vi "Shutdown.vi"(8 "error in (no error)":errorcluster, 11 "Stage_MadCityLabMicro in":refnum<class "Stage_MadCityLabMicro.lvclass">) -> (0 "error out":errorcluster, 3 "Stage_MadCityLabMicro out":refnum<class "Stage_MadCityLabMicro.lvclass">)   [LabVIEW 2020, in "Stage_MadCityLabMicro.lvlib" / "Stage_MadCityLabMicro.lvclass"]
uses:
  Stage_MadCityLabMicro.lvclass
  Stage_MadCityLabMicro.lvclass/Stage_MadCityLabMicro.ctl
  Hardware Abstraction Layer/Component/Stage/Stage/Stage.lvclass
  Dependency/MicroDrive.dll
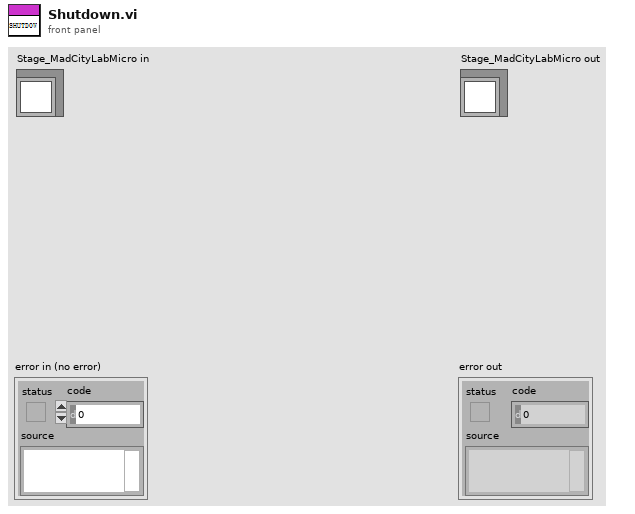
[diagram p1: front panel]
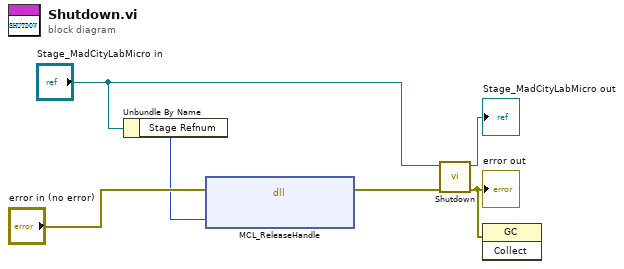
[diagram p0: block diagram]
diagram:
  n1 = Unbundle By Name("Stage_MadCityLabMicro in") -> ("Stage Refnum"=w1:i32)
  n2 = dll-call lib="E:/Development/DevHardSoftware/MicroscopyFramework/Model/Hardware Layer/Real Hardware/Stage_MadCityLabMicro/Stage_MadCityLabMicro/Dependency/MicroDrive.dll" fn="MCL_ReleaseHandle"(error in="error in (no error)", "handle"=w1) -> (error out=w4:errorcluster)  [unwired: 3 in, 2 out]
  n3 = call-parent "Shutdown.vi"("error in (no error)"=w4, "Device in"="Stage_MadCityLabMicro in") -> ("error out"=w6:errorcluster, "Device out"=→"Stage_MadCityLabMicro out":refnum<class "Stage_MadCityLabMicro.lvclass">)  [unwired: 8 in]
  "error out" <- w6
  n4 = invoke class="GC" method="Collect"(error in=w6) -> ()  [unwired: 2 in, 3 out]
